vi "CRYDIN-Loudness.vi"(0 "Ti-1":dbl[](array[numeric])) -> (7 "Ti":dbl[](array[numeric]))   [LabVIEW 2013]
panel:
  out "Numeric":dbl
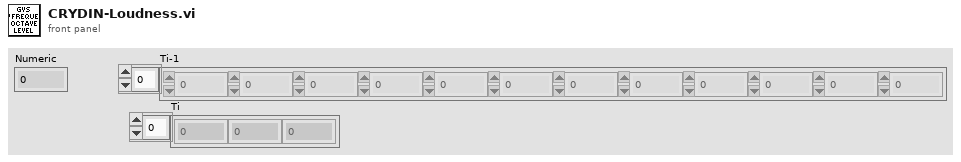
[diagram p1: front panel]
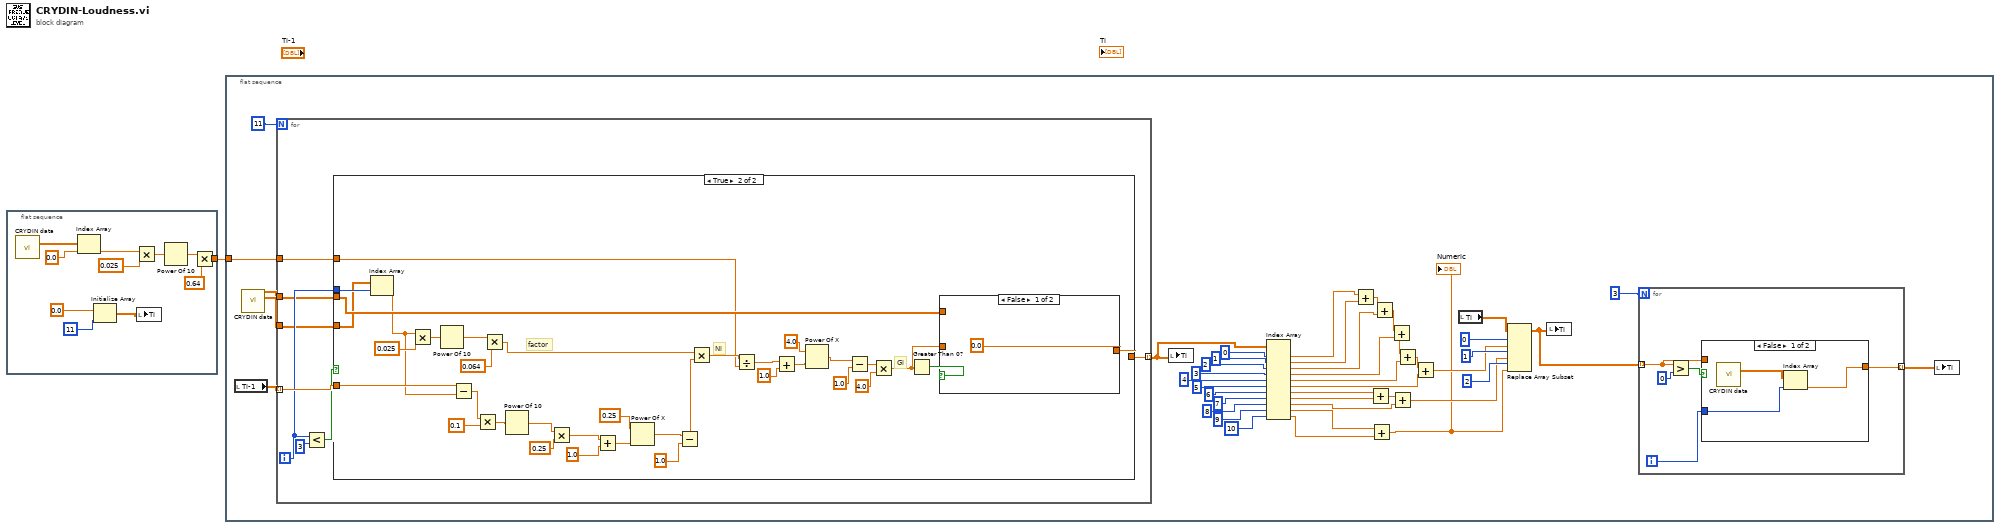
[diagram p0: block diagram]
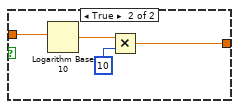
[diagram p2: hidden frame]
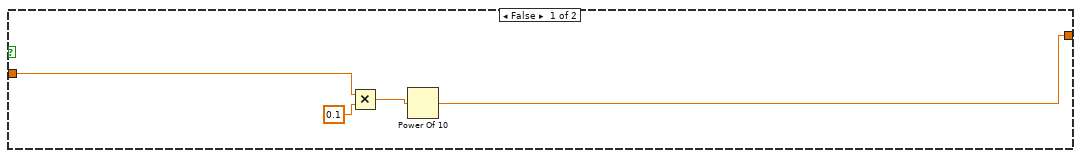
[diagram p3: hidden frame]
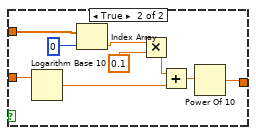
[diagram p4: hidden frame]
diagram:
  n1 = flat-sequence {
    tunnel: [w6] -> w1
    frame #0 {
      n2 = call "CRYDIN data.vi"() -> ("thresholdin quiet1"=w5:dbl[])  [unwired: 8 in, 7 out]
      n3 = Index Array(array=w5, index=0.0) -> (element=w10:dbl)
      n4 = Initialize Array(0.0, 11) -> (w4:dbl[])
      n5 = Multiply(x=w10, y=0.025) -> (x*y=w11:dbl)
      n6 = local write "Ti"(w4) -> ()
      n7 = Power Of 10(x=w11) -> (10^x=w12:dbl)
      n8 = Multiply(x=w12, y=0.64) -> (x*y=w6:dbl)
    }
  }
  n9 = flat-sequence {
    tunnel: w1 -> [w21]
    frame #0 {
      n10 = local read "Ti-1"() -> (w13:dbl[])
      n11 = call "CRYDIN data.vi"() -> ("lowFrequeccy Threshold"=w22:dbl[], "thresholdin quiet1"=w23:dbl[])  [unwired: 8 in, 6 out]
      n12 = for {
        N: 11 -> [_]
        tunnel: w22 -> [w69]
        tunnel: w13 -> [w75] mode=indexing
        tunnel: [w74] -> w15 mode=indexing
        tunnel: w23 -> [w68]
        tunnel: w21 -> [w71]
        i -> [w70]
        n13 = Less?(x=w70, y=3) -> (x < y?=w72:bool)
        n14 = case shown="True" w72 {
          tunnel: w69 -> [_ w81]
          tunnel: w75 -> [w78 w85]
          tunnel: w68 -> [_ w84]
          tunnel: [w76 w86] -> w74
          tunnel: w71 -> [_ w83]
          tunnel: w70 -> [_ w82]
          frame False {
            n15 = Multiply(x=w78, y=0.1) -> (x*y=w77:dbl)
            n16 = Power Of 10(x=w77) -> (10^x=w76:dbl)
          }
          frame True {
            # "Gi"
            # "Ni"
            # "factor"
            n17 = Index Array(array=w81, index=w82) -> (element=w80:dbl)
            n18 = Multiply(x=w80, y=0.025) -> (x*y=w112:dbl)
            n19 = Power Of 10(x=w112) -> (10^x=w111:dbl)
            n20 = Subtract(x=w85, y=w80) -> (x-y=w109:dbl)
            n21 = Multiply(x=w109, y=0.1) -> (x*y=w108:dbl)
            n22 = Multiply(x=w111, y=0.064) -> (x*y=w99:dbl)
            n23 = Power Of 10(x=w108) -> (10^x=w107:dbl)
            n24 = Multiply(x=w107, y=0.25) -> (x*y=w105:dbl)
            n25 = Add(x=w105, y=1.0) -> (x+y=w103:dbl)
            n26 = Power Of X(1:w103, 2:0.25) -> (0:w101:dbl)
            n27 = Subtract(x=w101, y=1.0) -> (x-y=w98:dbl)
            n28 = Multiply(x=w99, y=w98) -> (x*y=w97:dbl)
            n29 = Divide(x=w97, y=w83) -> (x/y=w96:dbl)
            n30 = Add(x=w96, y=1.0) -> (x+y=w94:dbl)
            n31 = Power Of X(1:w94, 2:4.0) -> (0:w91:dbl)
            n32 = Subtract(x=w91, y=1.0) -> (x-y=w90:dbl)
            n33 = Multiply(x=w90, y=4.0) -> (x*y=w87:dbl)
            n34 = Greater Than 0?(x=w87) -> (x > 0?=w88:bool)
            n35 = case shown="False" w88 {
              tunnel: w87 -> [_ w124]
              tunnel: w84 -> [_ w123]
              tunnel: [0.0 w116] -> w86
              frame False {
              }
              frame True {
                n36 = Logarithm Base 10(1:w124) -> (0:w119:dbl)
                n37 = Index Array(array=w123, index=0) -> (element=w120:dbl)
                n38 = Multiply(x=w120, y=0.1) -> (x*y=w118:dbl)
                n39 = Add(x=w118, y=w119) -> (x+y=w117:dbl)
                n40 = Power Of 10(x=w117) -> (10^x=w116:dbl)
              }
            }
          }
        }
      }
      n41 = local write "Ti"(w15) -> ()
      n42 = Index Array(array=w15, index #1=0, index #2=1, index #3=2, index #4=3, index #5=4, index #6=5, index #7=6, index #8=7, index #9=8, index #10=9, index #11=10) -> (element #1=w43:dbl, element #2=w42:dbl, element #3=w40:dbl, element #4=w38:dbl, element #5=w37:dbl, element #6=w35:dbl, element #7=w33:dbl, element #8=w32:dbl, element #9=w31:dbl, element #10=w29:dbl, element #11=w28:dbl)
      n43 = Add(x=w43, y=w42) -> (x+y=w41:dbl)
      n44 = Add(x=w33, y=w32) -> (x+y=w30:dbl)
      n45 = Add(x=w29, y=w28) -> (x+y=w18:dbl)
      "Numeric" <- w18
      n46 = Add(x=w41, y=w40) -> (x+y=w39:dbl)
      n47 = Add(x=w39, y=w38) -> (x+y=w36:dbl)
      n48 = Add(x=w30, y=w31) -> (x+y=w19:dbl)
      n49 = Add(x=w36, y=w37) -> (x+y=w34:dbl)
      n50 = Add(x=w34, y=w35) -> (x+y=w20:dbl)
      n51 = local read "Ti"() -> (w17:dbl[])
      n52 = Replace Array Subset(array=w17, new element #1=w20, index #1=0, new element #2=w19, index #2=1, new element #3=w18, index #3=2) -> (w16:dbl[])
      n53 = local write "Ti"(w16) -> ()
      n54 = for {
        N: 3 -> [_]
        tunnel: w16 -> [w59] mode=indexing
        tunnel: [w58] -> w14 mode=indexing
        i -> [w57]
        n55 = Greater?(x=w59, y=0) -> (0:w56:bool)
        n56 = case shown="False" w56 {
          tunnel: w59 -> [_ w67]
          tunnel: [w61 w64] -> w58
          tunnel: w57 -> [w62 _]
          frame False {
            n57 = call "CRYDIN data.vi"() -> ("thresholdin quiet1"=w63:dbl[])  [unwired: 8 in, 7 out]
            n58 = Index Array(array=w63, index=w62) -> (element=w61:dbl)
          }
          frame True {
            n59 = Logarithm Base 10(1:w67) -> (0:w66:dbl)
            n60 = Multiply(x=w66, y=10) -> (x*y=w64:dbl)
          }
        }
      }
      n61 = local write "Ti"(w14) -> ()
    }
  }
